vi "Close.vi"(8 "error in":errorcluster, 11 "Control Mode in":refnum<class "Control Mode.lvclass">) -> (0 "error out":errorcluster, 3 "Control Mode out":refnum<class "Control Mode.lvclass">)   [LabVIEW 2023, in "Control Mode.lvclass"]
uses:
  Control Mode.lvclass
  Control Mode.lvclass/Control Mode.ctl
  <vilib>/ADAS Replay HIL/AdasHilServices/AdasHilChannelServices.lvlib
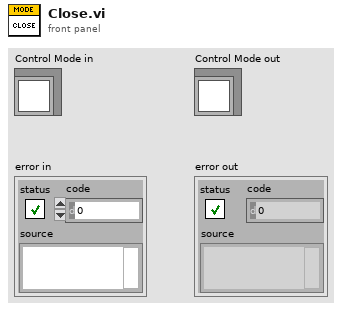
[diagram p1: front panel]
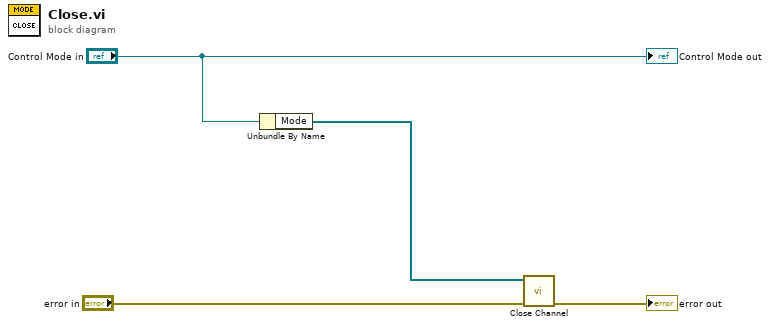
[diagram p0: block diagram]
diagram:
  n1 = Unbundle By Name("Control Mode in") -> ("Mode"=w1:refnum<k21>[])
  n2 = call <vilib>:"Close Channel.vi"("error in"="error in", "ADAS HIL Channel"=w1) -> ("error out"=→"error out":errorcluster)  [unwired: 9 in]
  "Control Mode out" <- "Control Mode in"
